vi "LogWriteError.vi"(8 "error constant":errorcluster, 11 "in string":string) -> ()   [LabVIEW 2019]
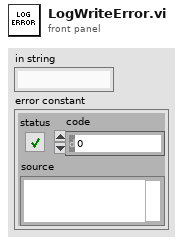
[diagram p1: front panel]
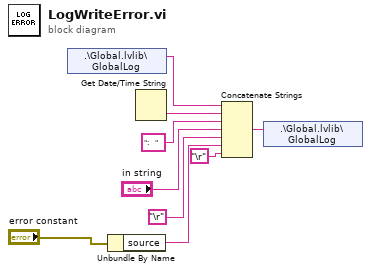
[diagram p0: block diagram]
diagram:
  n1 = shared-variable ".\\Global.lvlib\\GlobalLog"() -> (w3:string)  [unwired: 1 in, 1 out]
  n2 = Unbundle By Name("error constant") -> ("source"=w5:string)
  n3 = Get Date/Time String() -> (time string=w2:string)  [unwired: 3 in, 1 out]
  n4 = Concatenate Strings(w3, w2, ":   " ("string"), "in string", "\r", w5, "\r") -> (w8:string)
  n5 = shared-variable ".\\Global.lvlib\\GlobalLog"(w8) -> ()  [unwired: 1 in, 1 out]
